vi "Test Process Wait For Lifecycle State While Clearing Throws Error.vi"(8 "error in (no error)":errorcluster, 11 "Process Test In":refnum<class "Process Test.lvclass">) -> (0 "error out":errorcluster, 3 "Process Test Out":refnum<class "Process Test.lvclass">)   [LabVIEW 2020, in "Process Test.lvclass"]
uses:
  Process Test.lvclass
  Framework/Process/Process.lvclass
  <vilib>/Asteme/LUnit/Test Case.lvclass
  Framework/Process/Public/Lifecycle/Lifecycle State.ctl
  Support/Framework Test Support.lvlib
  C:/Users/anton/Documents/GitHub/Triarc-Framework/source/Framework Test/Base Class Test/Base Test.lvclass
  C:/Program Files (x86)/National Instruments/LabVIEW 2020/vi.lib/Asteme/LUnit/Test Case.lvclass
  C:/Users/anton/Documents/GitHub/Triarc-Framework/source/Framework Test/Process Test/Process Test.lvclass
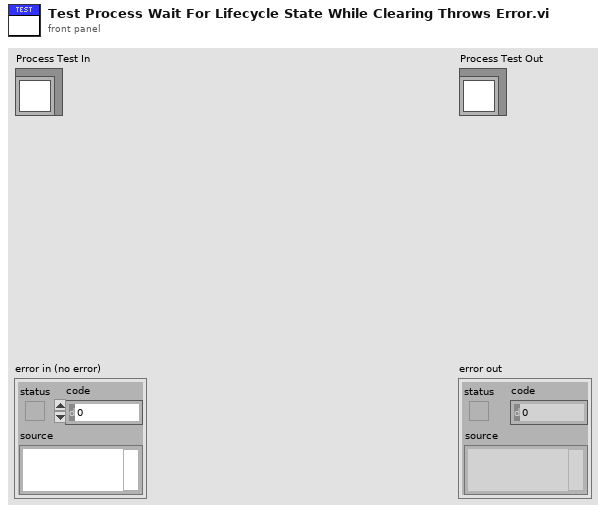
[diagram p1: front panel]
types:
  T1 = typedef "Process.lvclass/Lifecycle State.ctl" = enum16{"Uninitialized", "Initialized", "Started", "Running", "Stopped", "Finished"}
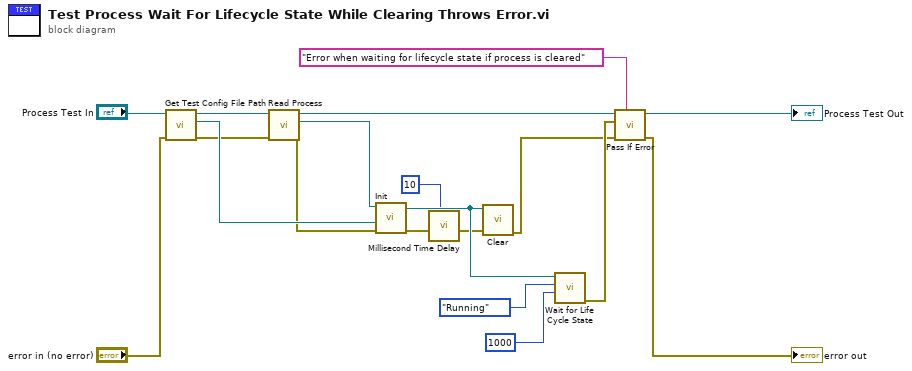
[diagram p0: block diagram]
diagram:
  n1 = call-dynamic "Get Test Config File Path.vi"("error in (no error)"="error in (no error)", "Base Class Test in"="Process Test In") -> ("error out"=w12:errorcluster, "Test config path"=w15:path, "Base Class Test out"=w17:refnum<class "Process Test.lvclass">)  [unwired: 7 in]
  n2 = call "Read Process.vi"("error in (no error)"=w12, "Process Test in"=w17) -> ("error out"=w13:errorcluster, "Process.lvclass"=w14:refnum<class "Process.lvclass">, "Process Test out"=w8:refnum<class "Process Test.lvclass">)  [unwired: 7 in]
  n3 = call-dynamic "Init.vi"("error in (no error)"=w13, "Config File Path"=w15, "Process In"=w14) -> ("error out"=w18:errorcluster, "Process Out"=w11:refnum<class "Process.lvclass">)  [unwired: 7 in]
  n4 = call "Millisecond Time Delay.vi"("milliseconds to wait"=u32 10, "error in (no error)"=w18) -> ("error out"=w2:errorcluster)  [unwired: 7 in]
  n5 = call-dynamic "Clear.vi"("error in (no error)"=w2, "Process In"=w11) -> ("error out"=w3:errorcluster)  [unwired: 9 in]
  n6 = call "Wait for Life Cycle State.vi"("timeout in ms (-1)"=1000, "Lifecycle State"=Lifecycle_State."Running", "Process In"=w11) -> ("error out"=w10:errorcluster)  [unwired: 6 in, 2 out]
  n7 = call <vilib>:"Pass If Error.vi"("Description"="Error when waiting for lifecycle state if process is cleared", "error in (no error)"=w3, "Assert error"=w10, "Test Case In"=w8) -> ("error out"=→"error out":errorcluster, "Test Case Out"=→"Process Test Out":refnum<class "Process Test.lvclass">)  [unwired: 6 in]
